vi "Calculate S21 S12 phase.vi"(0 "S Parameters in":cdb[][](array[numeric]), 5 "Frequencies":dbl[](array[numeric]), 11 "error in (no error)":errorcluster) -> (4 "S Parameters out":cdb[][](array[numeric]), 15 "error out":errorcluster)   [LabVIEW 2023, in "RFFixtureCharact.Public.lvlib" / "Vector Abstract Path.lvclass"]
uses:
  Vector Abstract Path.lvclass
  Vector Abstract Path.lvclass/Vector Abstract Path.ctl
  <vilib>/Analysis/NI_AALPro.lvlib
  Common/RFCalAndFixtureCharact.Common.lvlib
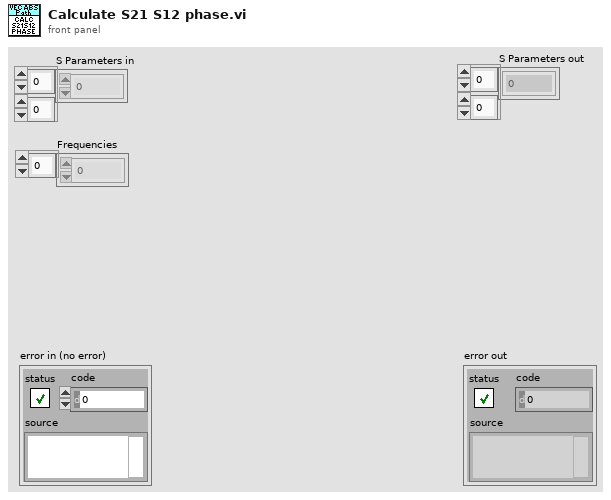
[diagram p1: front panel]
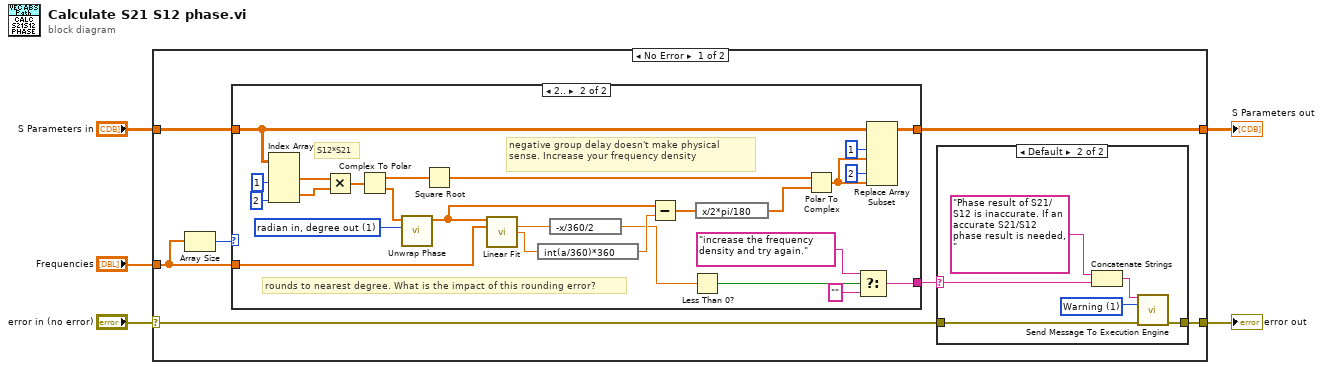
[diagram p0: block diagram]
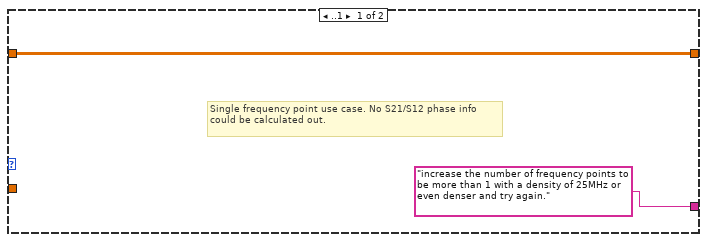
[diagram p3: hidden frame]
diagram:
  n1 = case shown="No Error" "error in (no error)" {
    selector: "error in (no error)" -> [w7 w49]
    tunnel: "S Parameters in" -> [w12 w48]
    tunnel: "Frequencies" -> [w9 _]
    tunnel: [w8 w49] -> w4
    tunnel: [w11 w48] -> w1
    frame No Error {
      n2 = Array Size(array=w9) -> (size(s)=w10:i32)
      n3 = case shown="2.." w10 {
        tunnel: w9 -> [_ w39]
        tunnel: w12 -> [w21 w37]
        tunnel: [w21 w33] -> w11
        tunnel: ["increase the number of frequency points to be more than 1 with a density of 25MHz or even denser and try again." ("message") w24] -> w6
        frame ..1 {
          # "Single frequency point use case. No S21/S12 phase info could be calculated out."
        }
        frame 2.. {
          w43 = 1 items=["radian in, radian out", "radian in, degree out", "degree in, degree out", "degree in, radian out"] ("phase unit")
          # "negative group delay doesn't make physical sense. Increase your frequency density"
          # "rounds to nearest degree. What is the impact of this rounding error?"
          # "S12*S21"
          n4 = Index Array(array=w37, index (col) #1=1 ("index"), index (col) #2=2 ("index")) -> (element #1=w47:cdb[], element #2=w46:cdb[])  [unwired: 2 in]
          n5 = Multiply(x=w47, y=w46) -> (x*y=w45:cdb[])
          n6 = Complex To Polar(r * e^(i*theta)=w45) -> (r=w40:dbl[], theta=w44:dbl[])
          n7 = call <vilib>:"Unwrap Phase.vi"("phase unit"=w43, "Phase"=w44) -> ("Unwrapped Phase"=w30:dbl[])  [unwired: 8 in, 1 out]
          n8 = Square Root(x=w40) -> (sqrt(x)=w38:dbl[])
          n9 = call <vilib>:"Linear Fit.vi"("Y"=w30, "X"=w39) -> ("slope"=w32:dbl, "intercept"=w29:dbl)  [unwired: 9 in, 3 out]
          n10 = expression code="int(a/360)*360"(w29) -> (w27:dbl)
          n11 = expression code="-x/360/2"(w32) -> (w26:dbl)
          n12 = Subtract(x=w30, y=w27) -> (x-y=w28:dbl[])
          n13 = Less Than 0?(x=w26) -> (x < 0?=w25:bool)
          n14 = expression code="x/2*pi/180"(w28) -> (w31:dbl[])
          n15 = Polar To Complex(1:w31, 2:w38) -> (0:w35:cdb[])
          n16 = Select(t="increase the frequency density and try again." ("message"), s=w25, f="") -> (s? t:f=w24:string)
          n17 = Replace Array Subset(array=w37, new element #1=w35, index (col) #1=1 ("disabled index (col)"), new element #2=w35, index (col) #2=2 ("index (col)")) -> (w33:cdb[][])  [unwired: 2 in]
        }
      }
      n18 = case shown="Default" w6 {
        selector: w6 -> [_ w14]
        tunnel: [w13 w18] -> w8
        tunnel: w7 -> [w13 w17]
        frame "" {
        }
        frame Default {
          w19 = 1 items=["Info", "Warning", "Error"] ("messageType")
          n19 = Concatenate Strings("Phase result of S21/S12 is inaccurate. If an accurate S21/S12 phase result is needed, " ("message"), w14) -> (w15:string)
          n20 = call "Send Message To Execution Engine.vi"("Message"=w15, "Message Type"=w19, "error in (no error)"=w17) -> ("error out"=w18:errorcluster)  [unwired: 12 in]
        }
      }
    }
    frame Error {
    }
  }
  "error out" <- w4
  "S Parameters out" <- w1
